vi "stm_GetIDfromName.vi"(9 "Name":string, 11 "MetaData":T2[](array[typedef])) -> (1 "Found":bool, 3 "Meta ID":T1)   [LabVIEW 2015]
doc: "This VI looks up the Meta data index using the Meta data name."
uses:
  Data Def/stm_MetaElement.ctl
  Data Def/stm_MetaDataElement.ctl
  Data Def/stm_MetaID.ctl
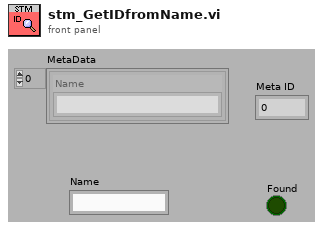
[diagram p1: front panel]
types:
  T1 = typedef "stm_MetaID.ctl" = u16
  T2 = typedef "stm_MetaElement.ctl" = cluster{"Name":T3}
  T3 = typedef "stm_MetaDataElement.ctl" = string
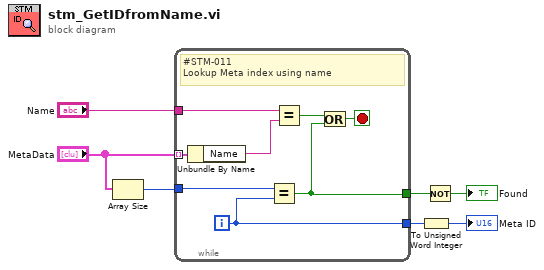
[diagram p0: block diagram]
diagram:
  n1 = Array Size(array="MetaData") -> (size(s)=w6:i32)
  n2 = while {
    tunnel: "MetaData" -> [w9] mode=indexing
    tunnel: w6 -> [w12]
    tunnel: "Name" -> [w15]
    tunnel: [w11] -> w2
    tunnel: [w10] -> w4
    i -> [w11]
    stop <- w13 stop-if-true
    # "#STM-011\nLookup Meta index using name"
    n3 = Unbundle By Name(w9) -> ("Name"=w8:T3)
    n4 = Equal?(x=w12, y=w11) -> (x = y?=w10:bool)
    n5 = Equal?(x=w15, y=w8) -> (x = y?=w14:bool)
    n6 = Or(x=w14, y=w10) -> (x .or. y?=w13:bool)
  }
  n7 = To Unsigned Word Integer(number=w2) -> (unsigned 16bit integer=→"Meta ID":u16)
  n8 = Not(x=w4) -> (.not. x?=→"Found":bool)
